vi "Close.vi"(8 "error in":errorcluster, 11 "IFGEN in":refnum<class "IGenerate Waveform.lvclass">) -> (0 "error out":errorcluster, 3 "IFGEN out":refnum<class "IGenerate Waveform.lvclass">)   [LabVIEW 2023, in "HAL Interfaces.lvlib" / "IGenerate Waveform.lvclass"]
uses:
  IGenerate Waveform.lvclass
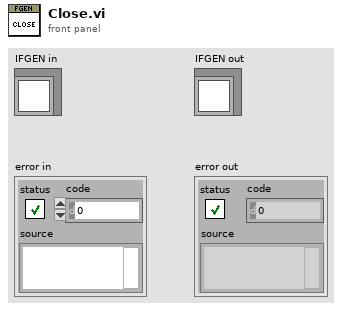
[diagram p1: front panel]
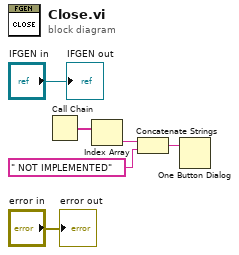
[diagram p0: block diagram]
diagram:
  n1 = Call Chain() -> (call chain=w4:string[])
  n2 = Index Array(array=w4) -> (element=w2:string)  [unwired: 1 in]
  n3 = Concatenate Strings(w2, " NOT IMPLEMENTED" ("string")) -> (w3:string)
  n4 = One Button Dialog(message=w3) -> ()  [unwired: 1 in, 1 out]
  "error out" <- "error in"
  "IFGEN out" <- "IFGEN in"
